vi "initialize_measurement.vi"(0 "Trigger\nmode":u32(ring) items=["Internal", "External"], 1 "Deprivation\nsettings":T3={"Frame Row"=0, "Kstd"=40.0, "# Images for\nsleep detection"=10, "Kmean"=1.5, "Start time of sleep detection (images):"=1000, "Column"=0, "Length (images)"=3600, "# TTL"=10000, "by x images after first detection"=0, "Between TTL pulses"=0, "\nby x detections"=9, "# Total immobility\n detections"=0.0, "max # adjacent\nTTL"=0, "TTL x start\ntime deprivation\n"=0, "Max #\nadjacent TTL"=10000, " Ca2+\nmode"=0} {"Column" items=["1", "2", "3", "4"]; "Frame Row" items=["1", "2", "3", "4"]}, 2 "Input\nparameters":T2={"Frame rate (ms)"=2000, "Worm Strain"="N2", "Time t"=0, "State"=enum."Image acquisition", "Acquisition time"=0.0, "Maximum # of images"=100000, "#TTL"=0, "time of third ttl "=100000, "ImSub Value"=0, "Time of last TTL"=0, "# Rows"=2, "# Columns"=2, "number of adjacentTTL"=0, "Sleep Deprivation status"="", "Sleep Detection"=FALSE, "Time of first sleep detection"=0, "# Sleep detections"=0, "Time max # adjacent TTL"=-10000, "Image t-1"=[], "Image t"=[]} {"# Columns" items=["1"=1, "2"=2, "3"=3, "4"=4]; "# Rows" items=["1"=1, "2"=2, "3"=3, "4"=4]}, 4 "Exposure \ntime":dbl=0.005 format="%.3f") -> (9 "Output\nparameters":T2={"Frame rate (ms)"=2000, "Worm Strain"="N2", "Time t"=0, "State"=enum."Image acquisition", "Acquisition time"=0.0, "Maximum # of images"=100000, "#TTL"=0, "time of third ttl "=100000, "ImSub Value"=0, "Time of last TTL"=0, "# Rows"=2, "# Columns"=2, "number of adjacentTTL"=0, "Sleep Deprivation status"="", "Sleep Detection"=FALSE, "Time of first sleep detection"=0, "# Sleep detections"=0, "Time max # adjacent TTL"=-10000, "Image t-1"=[], "Image t"=[]} {"# Columns" items=["1"=1, "2"=2, "3"=3, "4"=4]; "# Rows" items=["1"=1, "2"=2, "3"=3, "4"=4]})   [LabVIEW 2011]
uses:
  state.ctl
  Action Items.ctl
  Action-Init-Update-Get.ctl
panel:
  # "General settings"
  # "Select number of animals"
  # "Row"
  # "Column"
  # "General settings"
  # "Select number of animals"
  # "Row"
  # "Column"
  # "Sleep deprivation settings"
  # "Select deprivation animal"
  # "Row"
  # "Column"
  # "Sleep detection parameters"
  # "Sleep deprivation parameters"
  # "Delay deprivation start:"
  # "Pause deprivation (images):"
  # "Stop deprivation after:"
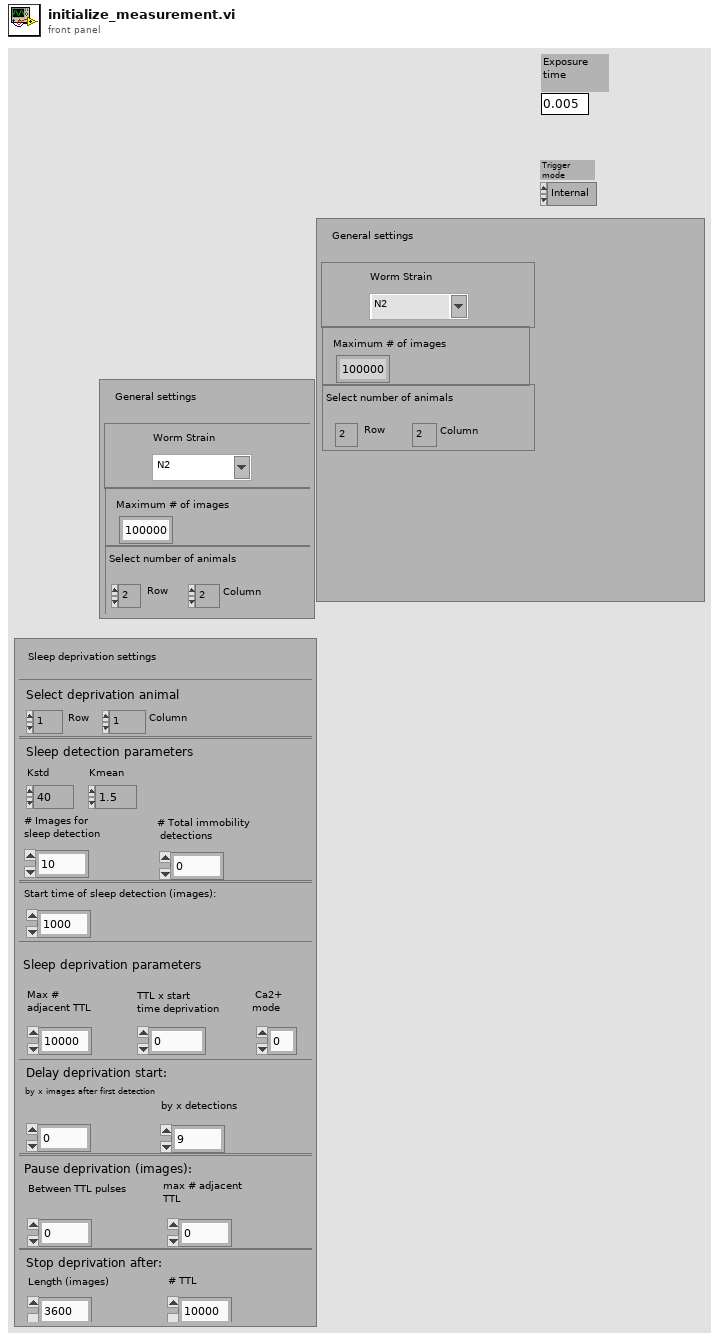
[diagram p1: front panel]
types:
  T1 = typedef "state.ctl" = enum16{"Initialize measurement", "Image acquisition", "Image processing", "Sleep detection", "Control TTL protocol ", "Sleep deprivation", "Update image & exit condition", "Wait "}
  T2 = cluster{"Frame rate (ms)":u32, "Worm Strain":string, "Time t":i32, "State":T1, "Acquisition time":dbl, "Maximum # of images":i32, "#TTL":i32, "time of third ttl ":i32, "ImSub Value":i32, "Time of last TTL":i32, "# Rows":u32, "# Columns":u32, "number of adjacentTTL":i32, "Sleep Deprivation status":string, "Sleep Detection":bool, "Time of first sleep detection":i32, "# Sleep detections":i32, "Time max # adjacent TTL":i32, "Image t-1":i32[][], "Image t":i32[][]}
  T3 = cluster{"Frame Row":u32, "Kstd":dbl, "# Images for\nsleep detection":i32, "Kmean":dbl, "Start time of sleep detection (images):":i32, "Column":u32, "Length (images)":i32, "# TTL":i32, "by x images after first detection":i32, "Between TTL pulses":i32, "\nby x detections":i32, "# Total immobility\n detections":dbl, "max # adjacent\nTTL":i32, "TTL x start\ntime deprivation\n":i32, "Max #\nadjacent TTL":i32, " Ca2+\nmode":i32}
  T4 = typedef "Action-Init-Update-Get.ctl" = enum16{"Initialize", "Update", "Get"}
  T5 = typedef "Action Items.ctl" = enum16{"Initialize", "Get"}
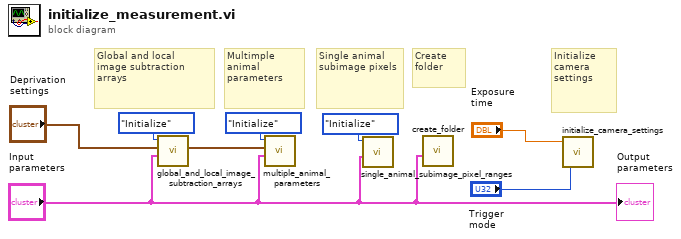
[diagram p0: block diagram]
diagram:
  # "Initialize\ncamera\nsettings"
  # "Global and local\nimage subtraction arrays"
  # "Multimple animal parameters"
  # "Create \nfolder"
  # "Single animal subimage pixels"
  n1 = call "global_and_local_image_subtraction_arrays.vi"("Input \nparameters"="Input\nparameters", "Deprivation\nparameters"="Deprivation\nsettings", "State"=Action-Init-Update-Get."Initialize" ("Action")) -> ()  [unwired: 8 in, 1 out]
  n2 = call "multiple_animal_parameters.vi"("Input \nparameters"="Input\nparameters", "Deprivation\nSettings"="Deprivation\nsettings", "Action"=Action_Items."Initialize") -> ()  [unwired: 8 in, 1 out]
  n3 = call "single_animal_subimage_pixel_ranges.vi"("Input \nparameters"="Input\nparameters", "Action"=Action_Items."Initialize") -> ()  [unwired: 9 in, 1 out]
  n4 = call "create_folder.vi"("Input \nparameters"="Input\nparameters") -> ()  [unwired: 11 in]
  n5 = call "initialize_camera_settings.vi"("Trigger"="Trigger\nmode", "Exposure \ntime (secs)"="Exposure \ntime") -> ()  [unwired: 3 in]
  "Output\nparameters" <- "Input\nparameters"
